vi "TaskStart.vi"(8 "error in (no error)":errorcluster, 11 "DAQ Hardware In":T1={"Task"="", "Max"=5.0, "min"=-5.0, "Samples Rate"=1000.0, "Channels"=[]} {"min" format="%0.2f"; "Max" format="%0.2f"}) -> (0 "error out":errorcluster, 3 "DAQ Hardware Out":T1={"Task"="", "Max"=5.0, "min"=-5.0, "Samples Rate"=1000.0, "Channels"=[]} {"min" format="%0.2f"; "Max" format="%0.2f"})   [LabVIEW 2014, in "NIDAQ.lvlib"]
uses:
  NIDAQ.lvlib
  DAQHardware.ctl
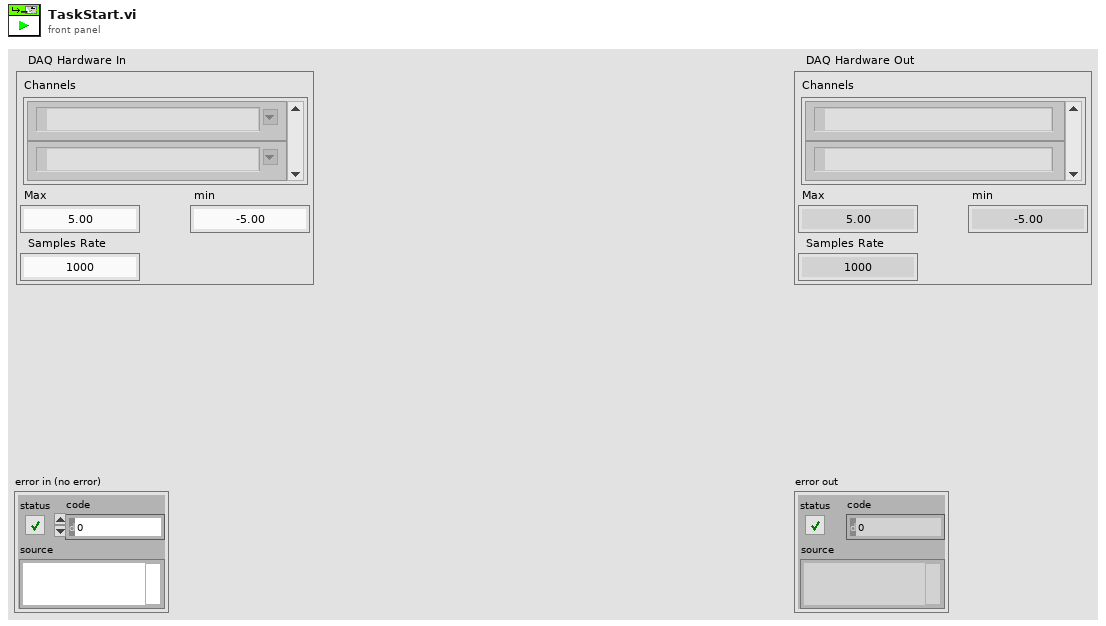
[diagram p1: front panel]
types:
  T1 = typedef "NIDAQ.lvlib/DAQHardware.ctl" = cluster{"Task":refnum<k21>, "Max":dbl, "min":dbl, "Samples Rate":dbl, "Channels":tag[]}
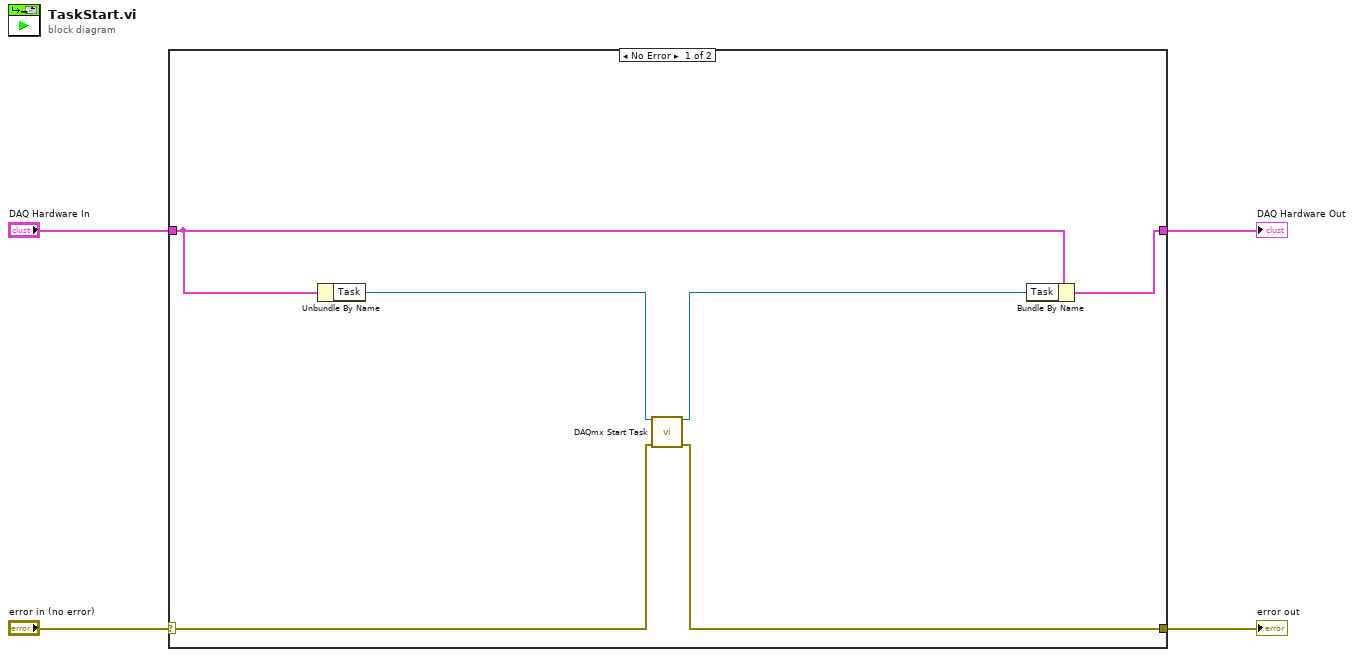
[diagram p0: block diagram]
diagram:
  n1 = case shown="No Error" "error in (no error)" {
    selector: "error in (no error)" -> [w7 w12]
    tunnel: [w8 w12] -> w3
    tunnel: "DAQ Hardware In" -> [w10 w11]
    tunnel: [w9 w11] -> w1
    frame No Error {
      n2 = Unbundle By Name(w10) -> ("Task"=w6:refnum<k21>)
      n3 = call <vilib>:"DAQmx Start Task.vi"("task/channels in"=w6, "error in"=w7) -> ("task out"=w5:refnum<k21>, "error out"=w8:errorcluster)  [unwired: 12 in]
      n4 = Bundle By Name(cluster=w10, "Task"=w5) -> (w9:T1)
    }
    frame Error {
    }
  }
  "error out" <- w3
  "DAQ Hardware Out" <- w1
